vi "Test_LogIfError_NoError_ErrorNotLogged.vi"(8 "error in (no error)":errorcluster, 11 "TestCase in":refnum<class "TestLocalLogInstance.lvclass">) -> (0 "error out":errorcluster, 3 "TestCase out":refnum<class "TestLocalLogInstance.lvclass">)   [LabVIEW 2017, in "TestLocalLogInstance.lvclass"]
uses:
  TestLocalLogInstance.lvclass
  Source/Composed Log/Types/Log Level.ctl
  Source/Composed Log/LoggerReference/LoggerReference.lvclass/LoggerReference.ctl
  Source/LVQueue Sink/LVQueue Sink.lvclass/LVQueue Sink.ctl
  f3a77fb9-85d9-428d-84c2-3a0191553ce9.vi
  Source/Composed Log/LoggerReference/Return Aggregate Queues.vi
  Source/Composed Log/LoggerReference/Add Aggregate Log.vi
  f3a77fb9-85d9-428d-84c2-3a0191553ce9.vi/84d13637-4ce7-4491-be04-10924981c3c8.vi
  Source/Composed Log/LoggerReference/Send Add Sink.vi
  Source/LVQueue Sink/LVQueue Sink.lvclass
  C:/CS/Internal/LabVIEW/Logger/Source/Composed Log/Log Sink/Log Sink.lvclass
  Source/Composed Log/Application Logger/Launch Worker Loop.vi
  Source/Composed Log/LoggerReference/Initialize Logger Instance.vi
  Source/Composed Log/LoggerReference/LoggerReference.lvclass
  Source/Composed Log/IErrorFormat/IErrorFormat.lvclass
  Source/Composed Log/Log Sink/Log Sink.lvclass
  <vilib>/addons/_JKI Toolkits/VI Tester/TestCase.llb/TestCase.lvclass
  Source/Composed Log/Composed Log.lvlib
  C:/Program Files (x86)/National Instruments/LabVIEW 2017/vi.lib/addons/_JKI Toolkits/VI Tester/TestCase.llb/TestCase.lvclass
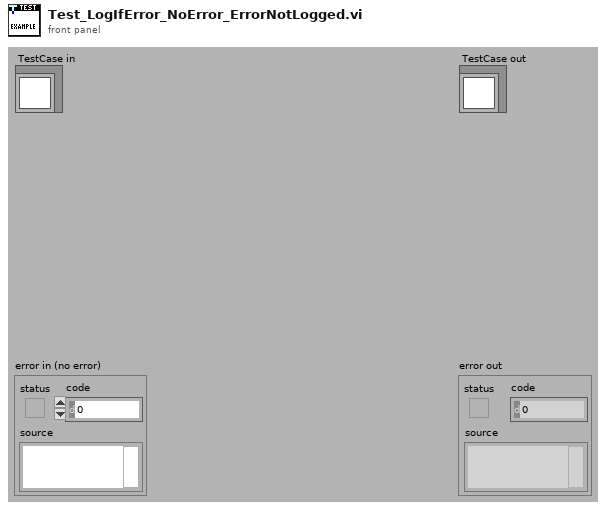
[diagram p1: front panel]
types:
  T1 = typedef "Composed Log.lvlib/Log Level.ctl" = enum16{"Debug", "Info", "Warning", "Error", "Critical"}
  T2 = typedef "Composed Log.lvlib/Log Packet.ctl" = cluster{"Data To Log":string, "Source":string, "Event Level":T1, "Event Time":timestamp}
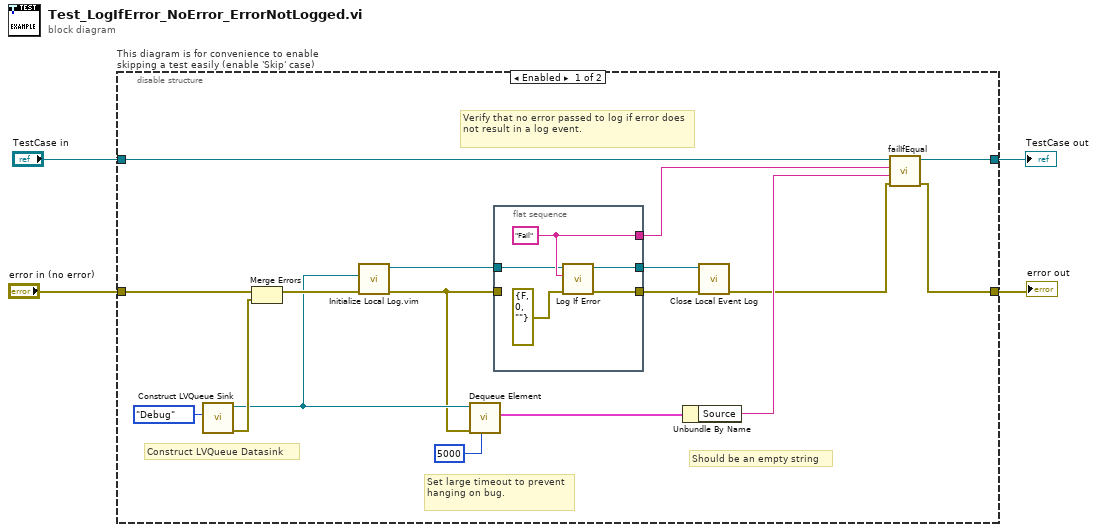
[diagram p0: block diagram]
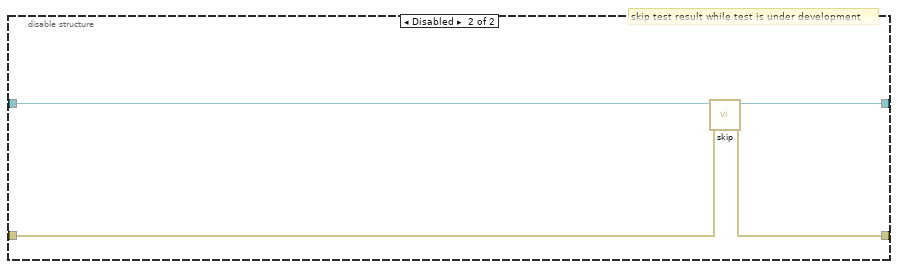
[diagram p2: hidden frame]
diagram:
  n1 = disable-structure "This diagram is for convenience to enable skipping a test easily (enable 'Skip' case)" shown="Enabled" {
    disable-tunnel: "TestCase in" -> [w15 w30]
    disable-tunnel: [w14 w28] -> w1
    disable-tunnel: [w16 w29] -> w3
    disable-tunnel: "error in (no error)" -> [w21 w27]
    frame Enabled {
      # "Should be an empty string"
      # "Construct LVQueue Datasink"
      # "Set large timeout to prevent hanging on bug."
      # "Verify that no error passed to log if error does not result in a log event."
      n2 = call "Construct LVQueue Sink.vi"("LogLevel"=Log_Level."Debug") -> ("error out"=w17:errorcluster, "LVQueue Sink out"=w10:refnum<class "LVQueue Sink.lvclass">)  [unwired: 9 in]
      n3 = Merge Errors(w21, w17) -> (w11:errorcluster)
      n4 = call "Initialize Local Log.vim"("error in (no error)"=w11, "Startup Sink(s)"=w10) -> ("error out"=w9:errorcluster, "Log Instance Reference"=w5:refnum<class "LoggerReference.lvclass">)  [unwired: 7 in, 1 out]
      n5 = call "Dequeue Element.vi"("timeout in ms (-1)"=5000, "error in (no error)"=w9, "LVQueue Sink in"=w10) -> ("Log Packet"=w18:T2)  [unwired: 5 in, 3 out]
      n6 = flat-sequence {
        tunnel: w9 -> [_]
        tunnel: [w26] -> w8
        tunnel: [w24] -> w12
        tunnel: [w23] -> w6
        tunnel: w5 -> [w22]
        frame #0 {
          w24 = "Fail" ("SourceID")
          n7 = call "Log If Error.vi"("Error In"=errorcluster {"status"=FALSE, "code"=0, "source"=""}, "SourceID"=w24, "Log Instance"=w22) -> ("error out"=w26:errorcluster, "Log Instance Out"=w23:refnum<class "LoggerReference.lvclass">)  [unwired: 7 in]
        }
      }
      n8 = Unbundle By Name(w18) -> ("Source"=w13:string)
      n9 = call "Close Local Event Log.vi"("error in (no error)"=w8, "Log Instance"=w6) -> ("error out"=w7:errorcluster)  [unwired: 9 in]
      n10 = call-dynamic "failIfEqual.vi"("error in (no error)"=w7, "y"=w13, "x"=w12, "TestCase in"=w15) -> ("error out"=w16:errorcluster, "TestCase out"=w14:refnum<class "TestLocalLogInstance.lvclass">)  [unwired: 6 in]
    }
    frame Disabled {
      # "skip test result while test is under development"
      n11 = call <vilib>:"skip.vi"("error in (no error)"=w27, "TestCase in"=w30) -> ("error out"=w29:errorcluster, "TestCase out"=w28:refnum<class "TestLocalLogInstance.lvclass">)  [unwired: 8 in]
    }
  }
  "error out" <- w3
  "TestCase out" <- w1
